vi "eV10_test.vi"() -> ()   [LabVIEW 2014]
panel:
  in  "eV10":bool
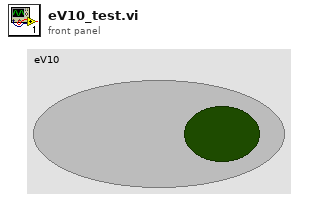
[diagram p1: front panel]
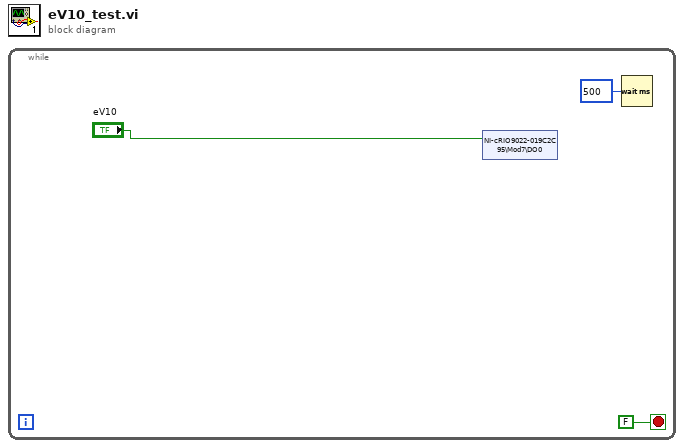
[diagram p0: block diagram]
diagram:
  n1 = while {
    stop <- FALSE stop-if-true
    n2 = shared-variable "NI-cRIO9022-019C2C95\\Mod7\\DO0"("eV10") -> ()  [unwired: 1 in, 1 out]
    n3 = Wait (ms)(milliseconds to wait=u32 500) -> ()  [unwired: 1 out]
  }
